vi "TestWriteOneSamp.vi"() -> ()   [LabVIEW 2014, in "FgenModule.lvlib"]
uses:
  FgenModule.lvlib
  FgenPlugins/NiPxi6733Class/NiPxi6733.lvclass
  FgenPlugins/FgenPluginBaseClass/FgenPluginsBase.lvclass/FgenPluginsBase.ctl
  FgenPlugins/FgenPluginBaseClass/Accessors/Read FunctionClass.vi
  FgenPlugins/FgenPluginBaseClass/Accessors/Read FunctionINIFilePath.vi
  MemberClasses/FunctionBaseClass/FunctionBase.lvclass
panel:
  in  "Path":path
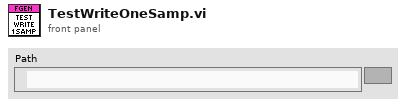
[diagram p1: front panel]
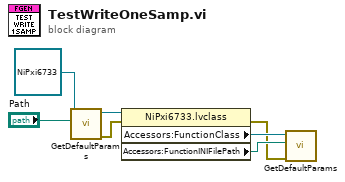
[diagram p0: block diagram]
diagram:
  n1 = call-dynamic "GetDefaultParams.vi"("Path"="Path", "NiPxi6733 in"=refnum<class "NiPxi6733.lvclass"> refnum) -> ("error out"=w1:errorcluster, "NiPxi6733 out"=w5:refnum<class "NiPxi6733.lvclass">)  [unwired: 8 in]
  n2 = property class="NiPxi6733.lvclass"(reference=w5, error in=w1) -> (error out=w2:errorcluster, "Accessors:FunctionClass"=w4:refnum<class "FunctionBase.lvclass">, "Accessors:FunctionINIFilePath"=w3:path)  [unwired: 1 out]
  n3 = call-dynamic "GetDefaultParams.vi"("error in (no error)"=w2, "Path"=w3, "FunctionBase in"=w4) -> ()  [unwired: 7 in, 2 out]
